vi "Write Parent Class Path.vi"(10 "Parent Class Path":path, 11 "Concrete Message Scripter in":refnum<class "Concrete Message Scripter.lvclass">) -> (3 "Concrete Message Scripter out":refnum<class "Concrete Message Scripter.lvclass">)   [LabVIEW 2020, in "Message Maker.lvlib" / "Concrete Message Scripter.lvclass"]
uses:
  Concrete Message Scripter.lvclass
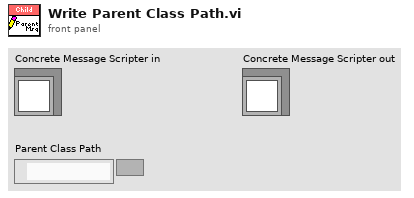
[diagram p1: front panel]
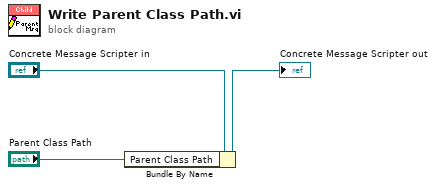
[diagram p0: block diagram]
diagram:
  n1 = Bundle By Name(cluster="Concrete Message Scripter in", "Parent Class Path"="Parent Class Path") -> (→"Concrete Message Scripter out":refnum<class "Concrete Message Scripter.lvclass">)
